vi "Generic Object Serializer Constant.vi"   [LabVIEW 2017]
doc: "Represents LabVIEW Objects as composite JSON Object. Parent classes form a union with their child classes."
uses:
  Generic Object Serializer/Generic Object Serializer.lvclass
  Generic Object Serializer/Type Name Handling.ctl
  Generic Object Serializer/Write Type Name Handling.vi
types:
  T1 = typedef "Generic Object Serializer.lvclass/Type Name Handling.ctl" = enum16{"None", "Inline"}
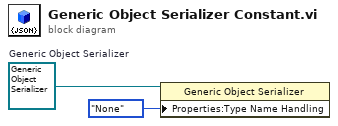
[diagram p0: block diagram]
diagram:
  w2 = refnum<class "Generic Object Serializer.lvclass"> refnum  # Generic Object Serializer
  n1 = property class="Generic Object Serializer"(reference=w2, "Properties:Type Name Handling"=Type_Name_Handling."None" ("Type Name Handling")) -> ()  [unwired: 1 in, 2 out]
